vi "Check Class Ancestry.vi"(1 "Class B":refnum<class>, 2 "Class A":refnum<class>) -> (0 "Is Class B a Descendant of Class A?":bool)   [LabVIEW 2020, in "Utilities.lvlib"]
doc: "Checks if Class B is a descendant of Class A. In other words, is Class B a child class of Class A?"
uses:
  Utilities.lvlib
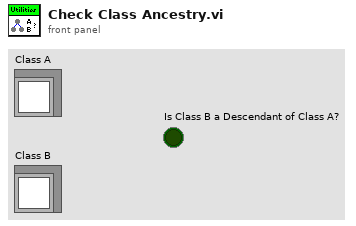
[diagram p1: front panel]
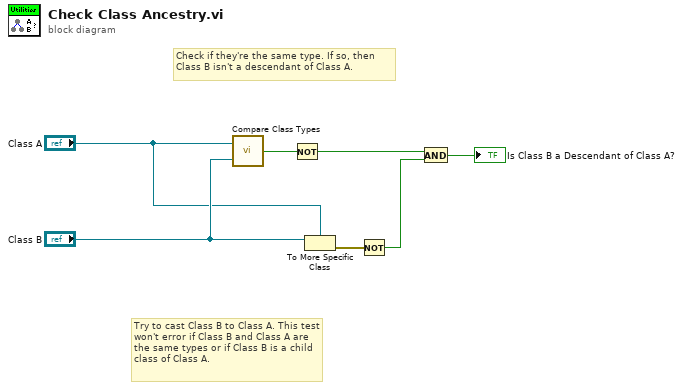
[diagram p0: block diagram]
diagram:
  # "Try to cast Class B to Class A. This test won't error if Class B and Class A are the same types or if Class B is a child class of Class A."
  # "Check if they're the same type. If so, then Class B isn't a descendant of Class A."
  n1 = call "Compare Class Types.vi"("Class B"="Class B", "Class A"="Class A") -> ("Class Types Equal?"=w5:bool)
  n2 = Not(x=w5) -> (.not. x?=w3:bool)
  n3 = To More Specific Class(target class="Class A", reference="Class B") -> (error out=w4:errorcluster)  [unwired: 1 in, 1 out]
  n4 = Not(x=w4) -> (.not. x?=w1:bool)
  n5 = And(x=w3, y=w1) -> (x .and. y?=→"Is Class B a Descendant of Class A?":bool)
